vi "VI Tree.vi"   [LabVIEW 2023, in "RTL-SDR.lvlib"]
uses:
  RTL-SDR.lvlib
  Initialize by Index.vi
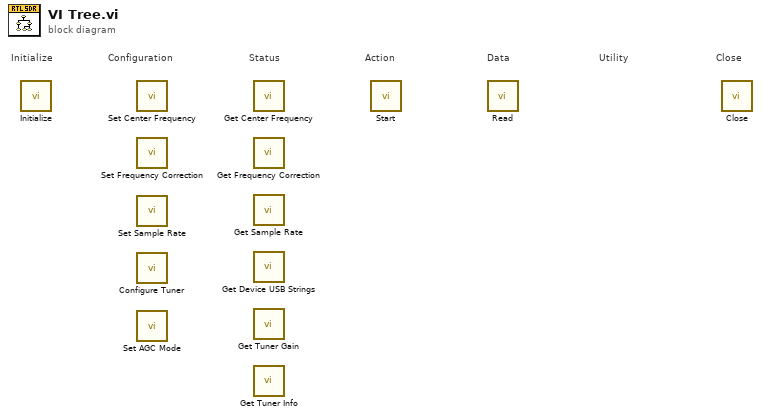
[diagram p0: block diagram]
diagram:
  # "Action"
  # "Utility"
  # "Data"
  # "Status"
  # "Configuration"
  # "Close"
  # "Initialize"
  n1 = call-poly "Initialize.vi"() -> ()  [unwired: 10 in, 2 out]
  n2 = call "Set Center Frequency.vi"() -> ()  [unwired: 10 in, 2 out]
  n3 = call "Set Frequency Correction.vi"() -> ()  [unwired: 10 in, 2 out]
  n4 = call "Set Sample Rate.vi"() -> ()  [unwired: 10 in, 2 out]
  n5 = call "Configure Tuner.vi"() -> ()  [unwired: 10 in, 2 out]
  n6 = call "Set AGC Mode.vi"() -> ()  [unwired: 10 in, 2 out]
  n7 = call "Get Center Frequency.vi"() -> ()  [unwired: 9 in, 3 out]
  n8 = call "Get Frequency Correction.vi"() -> ()  [unwired: 9 in, 3 out]
  n9 = call "Get Sample Rate.vi"() -> ()  [unwired: 9 in, 3 out]
  n10 = call "Get Device USB Strings.vi"() -> ()  [unwired: 8 in, 4 out]
  n11 = call "Get Tuner Gain.vi"() -> ()  [unwired: 9 in, 3 out]
  n12 = call "Get Tuner Info.vi"() -> ()  [unwired: 7 in, 5 out]
  n13 = call "Start.vi"() -> ()  [unwired: 10 in, 2 out]
  n14 = call "Read.vi"() -> ()  [unwired: 8 in, 4 out]
  n15 = call "Close.vi"() -> ()  [unwired: 11 in, 1 out]
